vi "Timeout.vi"(8 "error in":errorcluster, 11 "Modbus master in":refnum<class "Modbus Master.lvclass">) -> (0 "error out":errorcluster, 3 "Modbus master out":refnum<class "Modbus Master.lvclass">, 9 "Timer":u16, 10 "Temperature":u16)   [LabVIEW 2014, in "Files Library.lvlib"]
uses:
  Files Library.lvlib
  <vilib>/NI/Modbus Library/API/Master/Modbus Master.lvclass
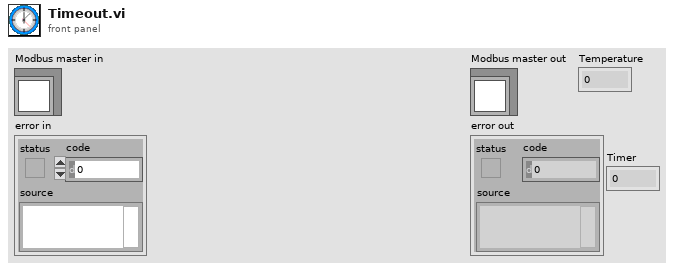
[diagram p1: front panel]
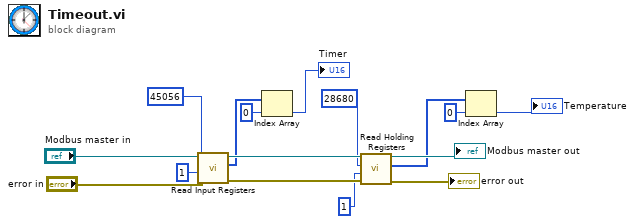
[diagram p0: block diagram]
diagram:
  n1 = call-dynamic "Read Input Registers.vi"("error in"="error in", "number of inputs"=u16 1, "starting address"=u16 45056, "Modbus master in"="Modbus master in") -> ("error out"=w11:errorcluster, "register values"=w6:u16[], "Modbus master out"=w12:refnum<class "Modbus Master.lvclass">)  [unwired: 5 in]
  n2 = Index Array(array=w6, index=0) -> (element=→"Timer":u16)
  n3 = call-dynamic "Read Holding Registers.vi"("error in"=w11, "number of inputs"=u16 1, "starting address"=u16 28680, "Modbus master in"=w12) -> ("error out"=→"error out":errorcluster, "register values"=w2:u16[], "Modbus master out"=→"Modbus master out":refnum<class "Modbus Master.lvclass">)  [unwired: 5 in]
  n4 = Index Array(array=w2, index=0) -> (element=→"Temperature":u16)
